vi "Real Inverse Matrix (LU).vi"(0 "A":T1) -> (1 "Inverse Matrix":T1, 2 "error":i32)   [LabVIEW 2018, in "NI_AALBase.lvlib"]
uses:
  <vilib>/Analysis/NI_AALBase.lvlib
  RealMatrix.ctl
  <resource>/lvanlys.dll
  NI_Matrix.lvlib
panel:
  # "Real Inverse Matrix (LU)"
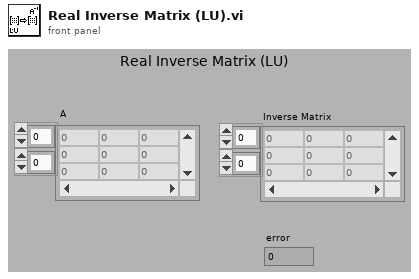
[diagram p1: front panel]
types:
  T1 = typedef "NI_Matrix.lvlib/RealMatrix.ctl" = dbl[][]
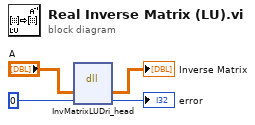
[diagram p0: block diagram]
diagram:
  n1 = dll-call lib="C:/Program Files (x86)/National Instruments/LabVIEW 2018/resource/lvanlys.*" fn="InvMatrixLUDri_head"("A"="A", "error"=0) -> ("A"=→"Inverse Matrix":T1, "error"=→"error":i32)  [unwired: 4 in, 2 out]
